vi "HW_Init_Serial_3.vi"(8 "error in":errorcluster, 9 "Acquisition FPS":T2, 10 "Close port? (F)":bool, 11 "VISA resource name":refnum<visa-resource-name>="Tracker") -> (0 "error out":errorcluster, 1 "FPS status":i32=80, 2 "Instrument OK?":bool, 3 "VISA resource name out":refnum<visa-resource-name>, 4 "Init status":T1={"VISA resource name"="", "FW version information"="0.0.0", "Sensor board size"="", "Sync mode status"="0", "FPS status"=0, "Instrument OK?"=FALSE})   [LabVIEW 2018, in "HW Interaction.lvlib"]
uses:
  HW Interaction.lvlib
  SubVi's/Controls/CTL_Acquisition_speed_selector.ctl
  Typedefs/CTL_HW_Init_outcome.ctl
  <vilib>/Utility/error.llb/DialogType.ctl
  Typedefs/CTL_HW_Init_internal_commands.ctl
  <vilib>/Instr/_visa.llb/VISA Set IO Buffer Mask.ctl
  <vilib>/Instr/_visa.llb/VISA Flush IO Buffer Mask.ctl
  <vilib>/Instr/_visa.llb/VISA Configure Serial Port (Instr).vi
  HW_Poll_Tracker_1.x.x.vi
  HW_Poll_Tracker_2.0.3.vi
  HW_Poll_Tracker_2.0.4+.vi
  Common_Resources.lvlib
panel:
  out "FPS setting VISA reply":string
  out "Poll Sync mode status":u32
  in  "FPS setup request":i32=80
  out "Poll Port data status":u32
  out "Port data status":i32=1
  out "Poll Binary":u32
  out "Poll Matrix":u32
  out "Poll Coord":u32
  out "Poll FPS":u32
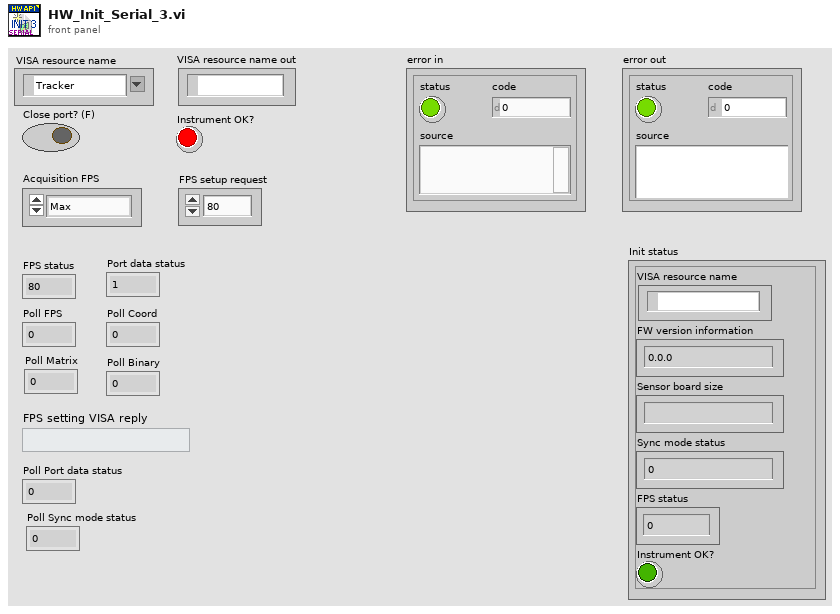
[diagram p1: front panel]
types:
  T1 = typedef "HW Interaction.lvlib/CTL_HW_Init_outcome.ctl" = cluster{"VISA resource name":refnum<visa-resource-name>, "FW version information":string, "Sensor board size":string, "Sync mode status":string, "FPS status":i32, "Instrument OK?":bool}
  T2 = typedef "Common_Resources.lvlib/CTL_Acquisition_speed_selector.ctl" = enum16{"Max", "Optimal", "Eco"}
  T3 = typedef "DialogType.ctl" = u16
  T4 = typedef "HW Interaction.lvlib/CTL_HW_Init_internal_commands.ctl" = cluster{"CMD":enum16{"None", "Exit", "Pause", "Step 1", "Step 2", "Step 3", "Step 4", "Step 5", "Step 6"}, "Payload":variant}
  T5 = enum16{"None", "Exit", "Pause", "Step 1", "Step 2", "Step 3", "Step 4"}
  T6 = enum16{"None", "Exit", "Pause", "Step 1", "Step 2", "Step 3", "Step 4", "Step 5", "Step 6"}
  T7 = typedef "VISA Flush IO Buffer Mask.ctl" = u16
  T8 = typedef "VISA Set IO Buffer Mask.ctl" = u16
  T9 = cluster{"Matrix mode status":string, "Coordinate mode status":string, "Binary mode status":string, "Sensors response":string, "FPS status":i32, "Port data status":i32}
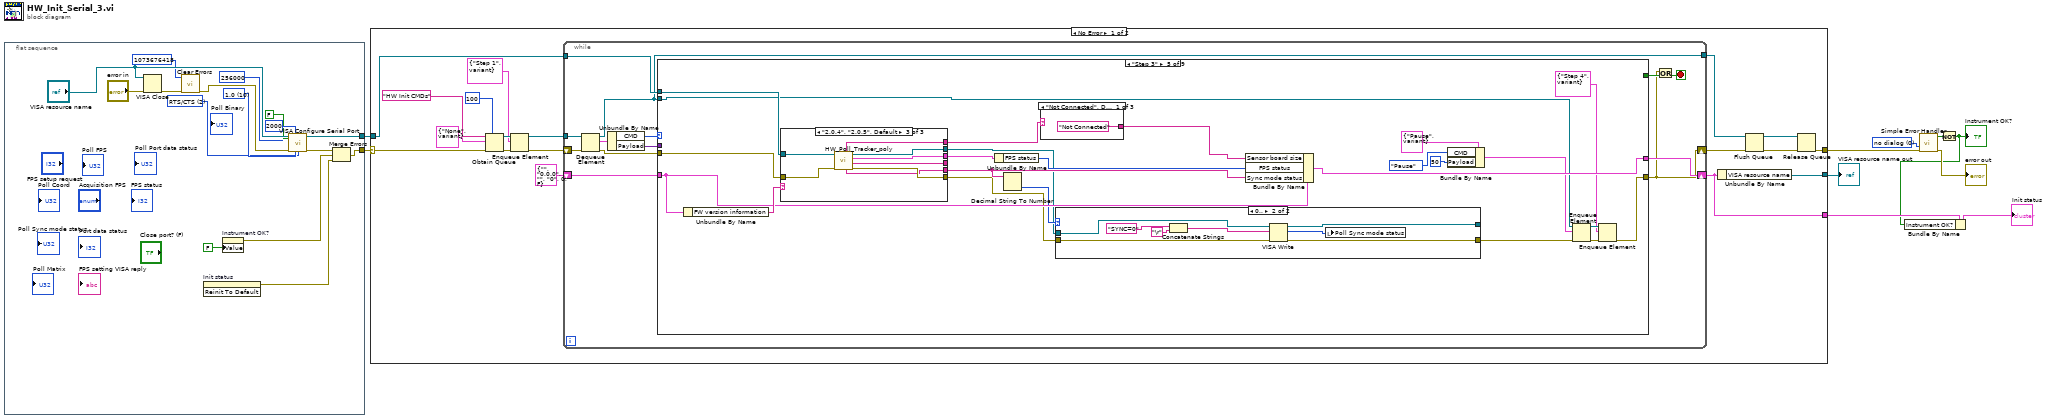
[diagram p0: block diagram]
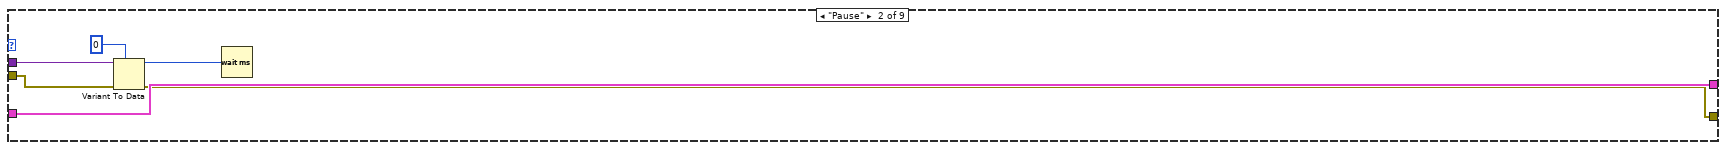
[diagram p3: hidden frame]
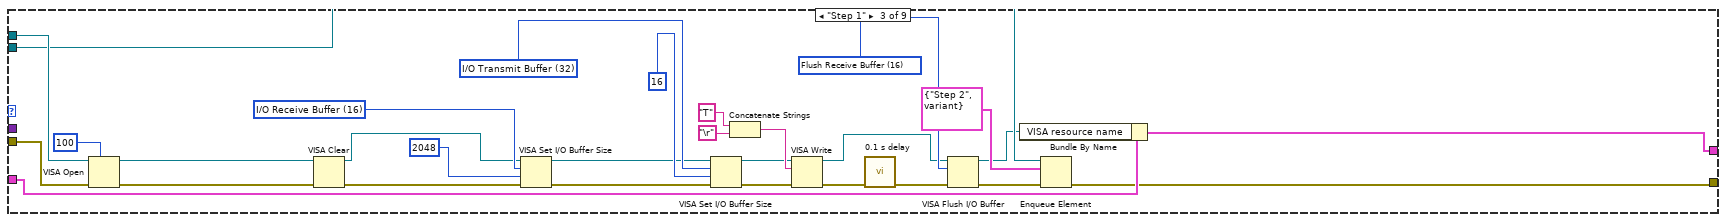
[diagram p4: hidden frame]
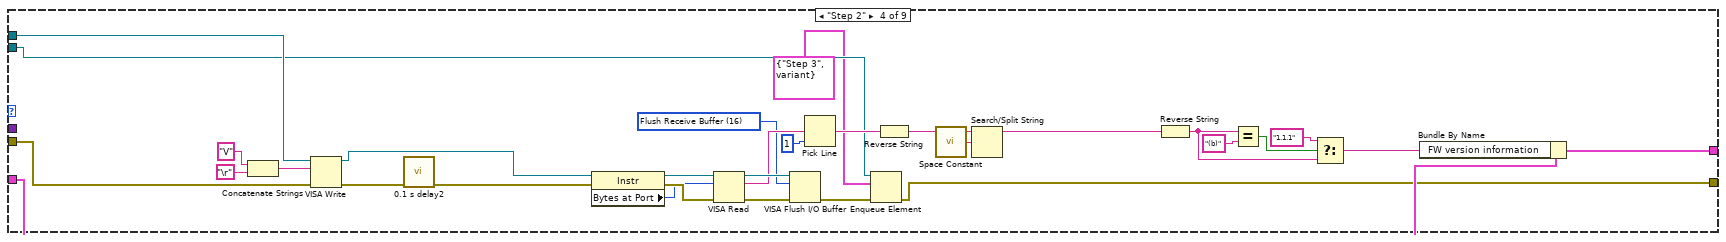
[diagram p5: hidden frame]
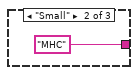
[diagram p6: hidden frame]
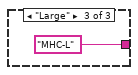
[diagram p7: hidden frame]
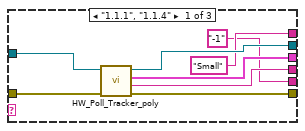
[diagram p9: hidden frame]
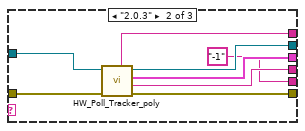
[diagram p10: hidden frame]
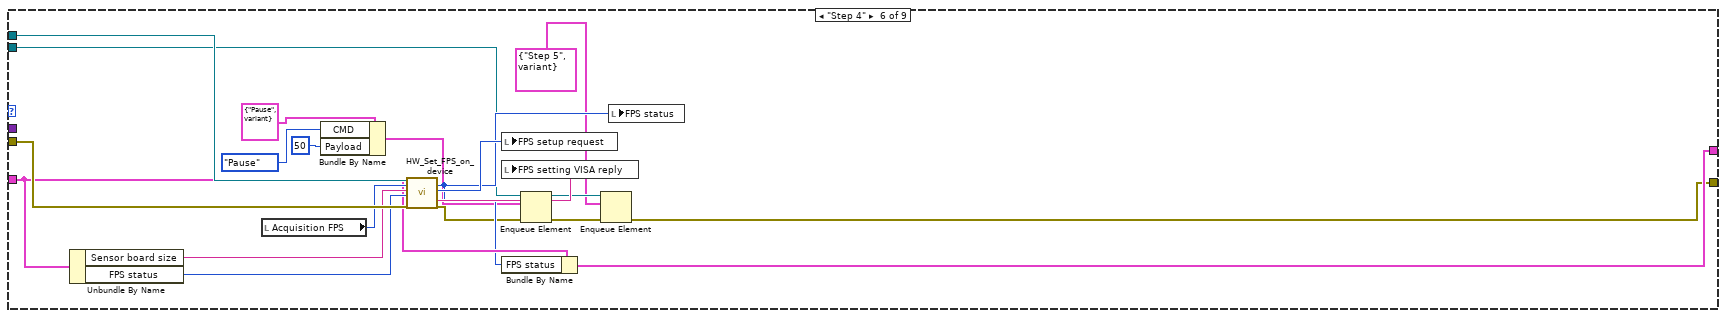
[diagram p11: hidden frame]
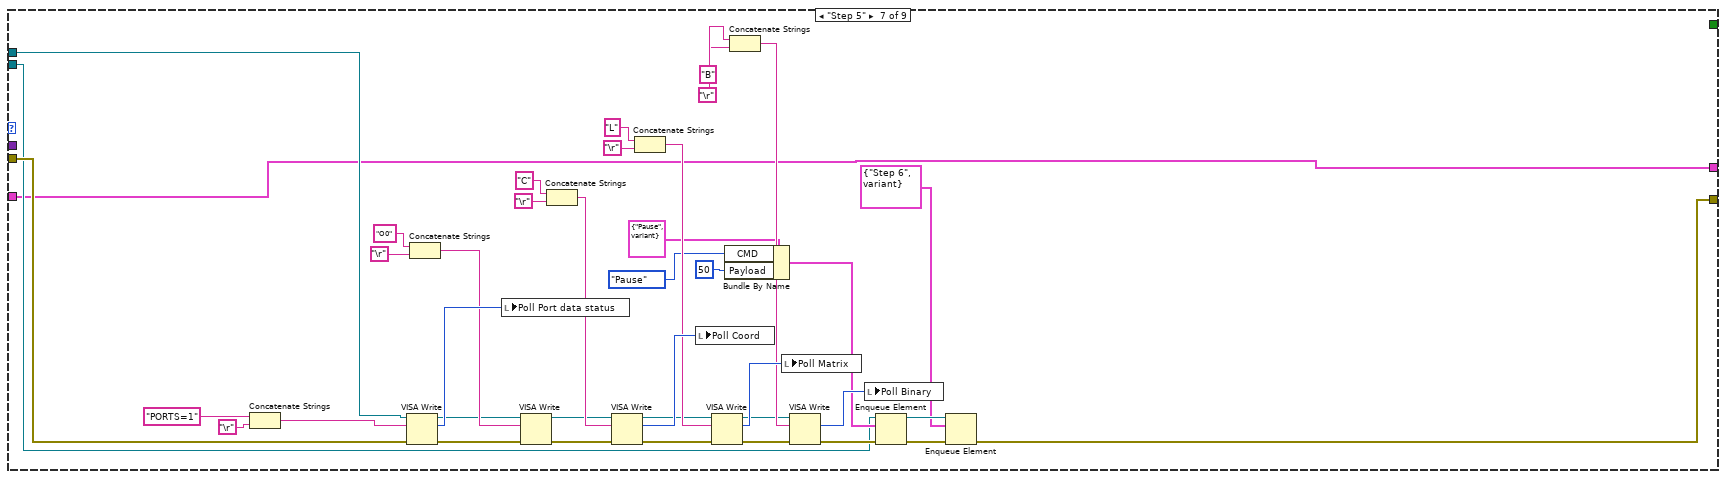
[diagram p12: hidden frame]
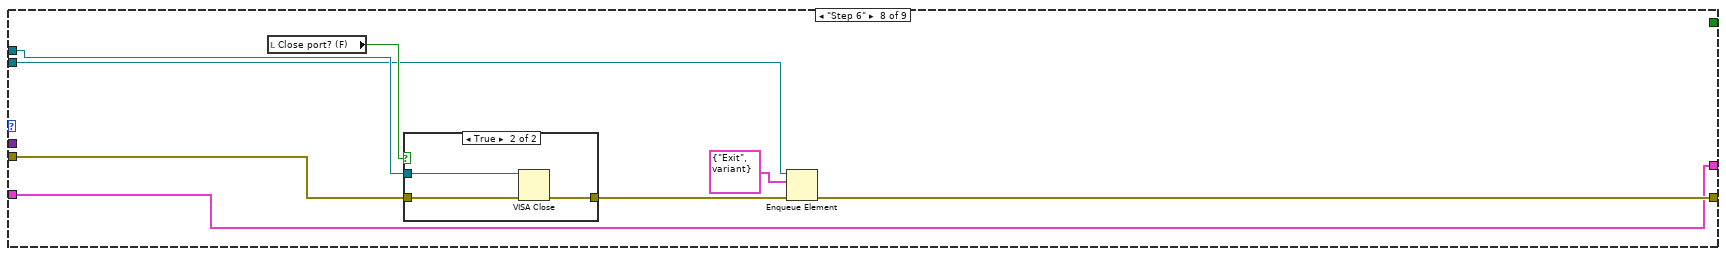
[diagram p13: hidden frame]
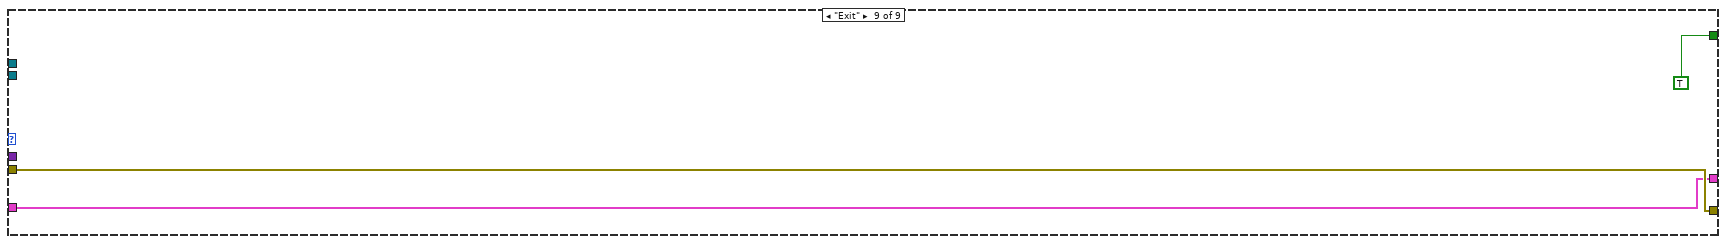
[diagram p15: hidden frame]
diagram:
  w9 = T3 0 items=["no dialog", "OK message", "continue or stop message", "OK message + warnings", "continue/stop + warnings"] ("type of dialog (OK msg:1)")
  n1 = flat-sequence {
    tunnel: [w16] -> w8
    tunnel: [w14] -> w7
    frame #0 {
      w18 = u16 10 items=["1.0"=10, "1.5"=15, "2.0"=20] ("stop bits (10: 1 bit)")
      w17 = u16 2 items=["None", "XON/XOFF", "RTS/CTS", "XON/XOFF & RTS/CTS", "DTR/DSR", "XON/XOFF & DTR/DSR"] ("flow control (0:none)")
      n2 = VISA Close(VISA resource name="VISA resource name", error in (no error)="error in") -> (error out=w24:errorcluster)
      n3 = call <vilib>:"Clear Errors.vi"("error in (no error)"=w24, "specific error code to clear (0: all)"=1073676418) -> ("error out"=w26:errorcluster)  [unwired: 4 in, 1 out]
      n4 = invoke on="Init status" class="Clust (strict)" method="Reinit To Default"() -> (error out=w11:errorcluster)  [unwired: 3 in, 2 out]
      n5 = property on="Instrument OK?" class="Bool (strict)"("Value"=FALSE ("Instrument OK?")) -> (error out=w12:errorcluster)  [unwired: 2 in, 1 out]
      n6 = call-poly "VISA Configure Serial Port"("VISA resource name"="VISA resource name", "timeout (10sec)"=u32 2000, "Enable Termination\nChar (T)"=FALSE ("Enable Termination\nChar (T)"), "baud rate (9600)"=u32 256000, "error in (no error)"=w26, "stop bits (10: 1 bit)"=w18, "flow control (0:none)"=w17) -> ("VISA resource name out"=w16:refnum<visa-resource-name>, "error out"=w15:errorcluster)  [unwired: 7 in]
      n7 = Merge Errors(w15, w12, w11) -> (w14:errorcluster)
    }
  }
  n8 = case shown="No Error" w7 {
    selector: w7 -> [w41 w261]
    tunnel: w8 -> [w44 w262]
    tunnel: [w29 w261] -> w6
    tunnel: [w28 _] -> w5
    tunnel: [w27 w262] -> w4
    frame No Error {
      n9 = Obtain Queue(max queue size (-1, unlimited)=100, name (unnamed)="HW Init CMDs", element data type=T4 {"CMD"=enum."None", "Payload"=variant} ("CMD and payload"), error in (no error)=w41) -> (queue out=w37:refnum<queue>, error out=w38:errorcluster)  [unwired: 1 in, 1 out]
      n10 = Enqueue Element(queue=w37, element=T4 {"CMD"=enum."Step 1", "Payload"=variant}, error in (no error)=w38) -> (queue out=w36:refnum<queue>, error out=w35:errorcluster)  [unwired: 1 in, 1 out]
      n11 = while {
        shift-right: [w45] -> w33
        shift-left: w35 -> [w53]
        tunnel: w44 -> [w56]
        shift-right: [w54] -> w28
        shift-left: T1 {"VISA resource name"="", "FW version information"="0.0.0", "Sensor board size"="", "Sync mode status"="0", "FPS status"=0, "Instrument OK?"=FALSE} ("Init status") -> [w55]
        tunnel: w36 -> [w51]
        tunnel: [w50] -> w32
        stop <- w46 stop-if-true
        n12 = Dequeue Element(queue=w51, error in (no error)=w53) -> (queue out=w50:refnum<queue>, element=w49:T4, error out=w52:errorcluster)  [unwired: 1 in, 1 out]
        n13 = Unbundle By Name(w49) -> ("CMD"=w48:T6, "Payload"=w47:variant)
        n14 = case shown="\"Step 3\"" w48 {
          tunnel: [_ _ _ _ _ _ _ _ TRUE] -> w57
          tunnel: w52 -> [w58 w63 w92 w122 w148 w205 w244 w252 w259]
          tunnel: w56 -> [_ _ w93 w121 w147 w204 w245 w251 _]
          tunnel: w55 -> [w59 w62 w72 w101 w145 w199 w206 w246 w258]
          tunnel: [w59 w62 w67 w99 w144 w198 w206 w246 w258] -> w54
          tunnel: w50 -> [_ _ w70 w97 w137 w195 w208 w250 _]
          tunnel: [w58 w61 w69 w96 w129 w187 w207 w247 w259] -> w45
          tunnel: w47 -> [_ w60 _ _ _ _ _ _ _]
          frame "None", Default {
          }
          frame "Pause" {
            n15 = Variant To Data(error in=w63, type=0, Variant=w60) -> (data=w64:i32, error out=w61:errorcluster)
            n16 = Wait (ms)(milliseconds to wait=w64) -> ()  [unwired: 1 out]
          }
          frame "Step 1" {
            w75 = T7 16 items=["Flush Receive Buffer"=16, "Write Transmit Buffer to Device"=32, "Flush Receive Buffer (No I/O)"=64, "Flush Transmit Buffer"=128] ("Mask")
            w85 = T8 32 items=["I/O Receive Buffer"=16, "I/O Transmit Buffer"=32, "I/O Receive and Transmit Buffer"=48] ("Mask")
            w89 = T8 16 items=["I/O Receive Buffer"=16, "I/O Transmit Buffer"=32, "I/O Receive and Transmit Buffer"=48] ("Mask")
            n17 = VISA Open(timeout (0)=u32 100 ("VISA Open timeout (0)"), error in (no error)=w92, VISA resource name=w93) -> (VISA resource name=w90:refnum<visa-resource-name>, error out=w91:errorcluster)  [unwired: 2 in]
            n18 = VISA Clear(VISA resource name=w90, error in (no error)=w91) -> (VISA resource name out=w86:refnum<visa-resource-name>, error out=w87:errorcluster)
            n19 = VISA Set I/O Buffer Size(VISA resource name=w86, mask (16)=w89, size (4096)=u32 2048, error in (no error)=w87) -> (VISA resource name out=w83:refnum<visa-resource-name>, error out=w82:errorcluster)
            n20 = VISA Set I/O Buffer Size(VISA resource name=w83, mask (16)=w85, size (4096)=u32 16, error in (no error)=w82) -> (VISA resource name out=w77:refnum<visa-resource-name>, error out=w78:errorcluster)
            n21 = Concatenate Strings("T" ("write buffer"), "\r") -> (w81:string)
            n22 = VISA Write(VISA resource name=w77, write buffer=w81, error in (no error)=w78) -> (VISA resource name out=w73:refnum<visa-resource-name>, error out=w76:errorcluster)  [unwired: 1 out]
            n23 = call "0.1 s delay"("error in (no error)"=w76) -> ("error out"=w74:errorcluster)  [unwired: 10 in]
            n24 = VISA Flush I/O Buffer(VISA resource name=w73, mask (16)=w75, error in (no error)=w74) -> (VISA resource name out=w66:refnum<visa-resource-name>, error out=w71:errorcluster)
            n25 = Bundle By Name(cluster=w72, "VISA resource name"=w66) -> (w67:T1)
            n26 = Enqueue Element(queue=w70, element=T4 {"CMD"=enum."Step 2", "Payload"=variant}, error in (no error)=w71) -> (error out=w69:errorcluster)  [unwired: 1 in, 2 out]
          }
          frame "Step 2" {
            w104 = T7 16 items=["Flush Receive Buffer"=16, "Write Transmit Buffer to Device"=32, "Flush Receive Buffer (No I/O)"=64, "Flush Transmit Buffer"=128] ("Mask")
            n27 = Concatenate Strings("V" ("write buffer"), "\r") -> (w125:string)
            n28 = VISA Write(VISA resource name=w121, write buffer=w125, error in (no error)=w122) -> (VISA resource name out=w103:refnum<visa-resource-name>, error out=w120:errorcluster)  [unwired: 1 out]
            n29 = call "0.1 s delay2"("error in (no error)"=w120) -> ("error out"=w102:errorcluster)  [unwired: 10 in]
            n30 = property class="Instr"(reference=w103, error in=w102) -> (reference out=w119:refnum<visa-resource-name>, error out=w118:errorcluster, "Bytes at Port"=w117:u32)
            n31 = VISA Read(VISA resource name=w119, byte count=w117, error in (no error)=w118) -> (VISA resource name out=w115:refnum<visa-resource-name>, read buffer=w114:string, error out=w116:errorcluster)  [unwired: 1 out]
            n32 = VISA Flush I/O Buffer(VISA resource name=w115, mask (16)=w104, error in (no error)=w116) -> (error out=w98:errorcluster)  [unwired: 1 out]
            n33 = Pick Line(multi-line string=w114, line index=1) -> (output string=w113:string)  [unwired: 1 in]
            n34 = Enqueue Element(queue=w97, element=T4 {"CMD"=enum."Step 3", "Payload"=variant}, error in (no error)=w98) -> (error out=w96:errorcluster)  [unwired: 1 in, 2 out]
            n35 = Reverse String(1:w113) -> (0:w112:string)
            n36 = call <vilib>:"Space Constant.vi"() -> ("String"=w111:string)
            n37 = Search/Split String(string=w112, search string/char (-)=w111) -> (substring before match=w110:string)  [unwired: 1 in, 2 out]
            n38 = Reverse String(1:w110) -> (0:w108:string)
            n39 = Equal?(x=w108, y="(b)") -> (x = y?=w109:bool)
            n40 = Select(t="1.1.1", s=w109, f=w108) -> (s? t:f=w100:string)
            n41 = Bundle By Name(cluster=w101, "FW version information"=w100) -> (w99:T1)
          }
          frame "Step 3" {
            n42 = Unbundle By Name(w145) -> ("FW version information"=w146:string)
            n43 = case shown="\"2.0.4\", \"2.0.5\", Default" w146 {
              tunnel: [w169 w174 w183] -> w139
              tunnel: [w168 w172 w180] -> _
              tunnel: w148 -> [w167 w177 w184]
              tunnel: w147 -> [w166 w175 w185]
              tunnel: [w165 w176 w179] -> w138
              tunnel: [w164 w173 w181] -> w143
              tunnel: ["Small" w171 w182] -> w127
              tunnel: ["-1" ("Sync mode status") "-1" ("Sync mode status") w178] -> w140
              frame "1.1.1", "1.1.4" {
                n44 = call-poly "HW_Poll_Tracker_poly.vi"("error in"=w167, "VISA resource name in"=w166) -> ("error out"=w165:errorcluster, "Read buffer"=w168:string, "Parameters output"=w164:T9, "VISA resource name out"=w169:refnum<visa-resource-name>)  [unwired: 6 in]
              }
              frame "2.0.3" {
                n45 = call-poly "HW_Poll_Tracker_poly.vi"("error in"=w177, "VISA resource name in"=w175) -> ("error out"=w176:errorcluster, "Read buffer"=w172:string, "Parameters output"=w173:T9, "VISA resource name out"=w174:refnum<visa-resource-name>, "Sensor board size"=w171:string)  [unwired: 5 in]
              }
              frame "2.0.4", "2.0.5", Default {
                n46 = call-poly "HW_Poll_Tracker_poly.vi"("error in"=w184, "VISA resource name in"=w185) -> ("error out"=w179:errorcluster, "Read buffer"=w180:string, "Parameters output"=w181:T9, "VISA resource name out"=w183:refnum<visa-resource-name>, "Sync mode status"=w178:string, "Sensor board size"=w182:string)  [unwired: 4 in]
              }
            }
            n47 = Unbundle By Name(w143) -> ("FPS status"=w142:i32)
            n48 = Decimal String To Number(string=w140) -> (number=w141:i32)  [unwired: 2 in, 1 out]
            n49 = case shown="\"Not Connected\", Default" w127 {
              tunnel: ["Not Connected" ("f") "MHC" ("x") "MHC-L" ("f")] -> w126
              frame "Not Connected", Default {
              }
              frame "Small" {
              }
              frame "Large" {
              }
            }
            n50 = case shown="0.." w141 {
              tunnel: w139 -> [w153 w160]
              tunnel: w138 -> [w152 w159]
              tunnel: [w152 w158] -> w136
              tunnel: [w153 w157] -> _
              frame -1, Default {
              }
              frame 0.. {
                n51 = Concatenate Strings("SYNC=0" ("write buffer"), "\r") -> (w161:string)
                n52 = VISA Write(VISA resource name=w160, write buffer=w161, error in (no error)=w159) -> (VISA resource name out=w157:refnum<visa-resource-name>, return count=w154:u32, error out=w158:errorcluster)
                n53 = local write "Poll Sync mode status"(w154) -> ()
              }
            }
            n54 = Bundle By Name(cluster=w145, "Sensor board size"=w126, "FPS status"=w142, "Sync mode status"=w140) -> (w144:T1)
            n55 = Bundle By Name(cluster=T4 {"CMD"=enum."Pause", "Payload"=variant} ("element"), "CMD"=T5."Pause", "Payload"=50) -> (w134:T4)
            n56 = Enqueue Element(queue=w137, element=w134, error in (no error)=w136) -> (queue out=w130:refnum<queue>, error out=w131:errorcluster)  [unwired: 1 in, 1 out]
            n57 = Enqueue Element(queue=w130, element=T4 {"CMD"=enum."Step 4", "Payload"=variant}, error in (no error)=w131) -> (error out=w129:errorcluster)  [unwired: 1 in, 2 out]
          }
          frame "Step 4" {
            n58 = Unbundle By Name(w199) -> ("Sensor board size"=w202:string, "FPS status"=w203:i32)
            n59 = local read "Acquisition FPS"() -> (w201:T2)
            n60 = Bundle By Name(cluster=T4 {"CMD"=enum."Pause", "Payload"=variant} ("element"), "CMD"=T5."Pause", "Payload"=50) -> (w190:T4)
            n61 = call "HW_Set_FPS_on_device.vi"("VISA in"=w204, "Desired FPS"=w201, "Sensor board size"=w202, "Current FPS"=w203, "Error in (no error)"=w205) -> ("FPS set on device"=w196:i32, "FPS requested"=w197:i32, "VISA reply"=w200:string, "Error out"=w194:errorcluster)  [unwired: 9 in, 2 out]
            n62 = local write "FPS setup request"(w197) -> ()
            n63 = local write "FPS setting VISA reply"(w200) -> ()
            n64 = Bundle By Name(cluster=w199, "FPS status"=w196) -> (w198:T1)
            n65 = Enqueue Element(queue=w195, element=w190, error in (no error)=w194) -> (queue out=w188:refnum<queue>, error out=w189:errorcluster)  [unwired: 1 in, 1 out]
            n66 = Enqueue Element(queue=w188, element=T4 {"CMD"=enum."Step 5", "Payload"=variant}, error in (no error)=w189) -> (error out=w187:errorcluster)  [unwired: 1 in, 2 out]
            n67 = local write "FPS status"(w196) -> ()
          }
          frame "Step 5" {
            n68 = Concatenate Strings("PORTS=1" ("write buffer"), "\r") -> (w241:string)
            n69 = VISA Write(VISA resource name=w245, write buffer=w241, error in (no error)=w244) -> (VISA resource name out=w235:refnum<visa-resource-name>, return count=w240:u32, error out=w236:errorcluster)
            n70 = Concatenate Strings("O0" ("write buffer"), "\r") -> (w239:string)
            n71 = local write "Poll Port data status"(w240) -> ()
            n72 = VISA Write(VISA resource name=w235, write buffer=w239, error in (no error)=w236) -> (VISA resource name out=w229:refnum<visa-resource-name>, error out=w230:errorcluster)  [unwired: 1 out]
            n73 = Concatenate Strings("C" ("write buffer"), "\r") -> (w233:string)
            n74 = VISA Write(VISA resource name=w229, write buffer=w233, error in (no error)=w230) -> (VISA resource name out=w223:refnum<visa-resource-name>, return count=w234:u32, error out=w224:errorcluster)
            n75 = Concatenate Strings("L" ("write buffer"), "\r") -> (w227:string)
            n76 = local write "Poll Coord"(w234) -> ()
            n77 = VISA Write(VISA resource name=w223, write buffer=w227, error in (no error)=w224) -> (VISA resource name out=w217:refnum<visa-resource-name>, return count=w228:u32, error out=w218:errorcluster)
            n78 = Bundle By Name(cluster=T4 {"CMD"=enum."Pause", "Payload"=variant} ("element"), "CMD"=T5."Pause", "Payload"=50) -> (w216:T4)
            n79 = Concatenate Strings("B" ("write buffer"), "\r") -> (w221:string)
            n80 = local write "Poll Matrix"(w228) -> ()
            n81 = VISA Write(VISA resource name=w217, write buffer=w221, error in (no error)=w218) -> (return count=w222:u32, error out=w209:errorcluster)  [unwired: 1 out]
            n82 = local write "Poll Binary"(w222) -> ()
            n83 = Enqueue Element(queue=w208, element=w216, error in (no error)=w209) -> (queue out=w214:refnum<queue>, error out=w215:errorcluster)  [unwired: 1 in, 1 out]
            n84 = Enqueue Element(queue=w214, element=T4 {"CMD"=enum."Step 6", "Payload"=variant}, error in (no error)=w215) -> (error out=w207:errorcluster)  [unwired: 1 in, 2 out]
          }
          frame "Step 6" {
            n85 = local read "Close port? (F)"() -> (w253:bool)
            n86 = case shown="True" w253 {
              tunnel: w252 -> [w254 w257]
              tunnel: [w254 w256] -> w249
              tunnel: w251 -> [_ w255]
              frame False {
              }
              frame True {
                n87 = VISA Close(VISA resource name=w255, error in (no error)=w257) -> (error out=w256:errorcluster)
              }
            }
            n88 = Enqueue Element(queue=w250, element=T4 {"CMD"=enum."Exit", "Payload"=variant}, error in (no error)=w249) -> (error out=w247:errorcluster)  [unwired: 1 in, 2 out]
          }
          frame "Exit" {
          }
        }
        n89 = Or(x=w45, y=w57) -> (x .or. y?=w46:bool)
      }
      n90 = Unbundle By Name(w28) -> ("VISA resource name"=w27:refnum<visa-resource-name>)
      n91 = Flush Queue(queue=w32, error in (no error)=w33) -> (queue out=w30:refnum<queue>, error out=w31:errorcluster)  [unwired: 1 out]
      n92 = Release Queue(queue=w30, error in (no error)=w31) -> (error out=w29:errorcluster)  [unwired: 1 in, 2 out]
    }
    frame Error {
    }
  }
  "VISA resource name out" <- w4
  n93 = call <vilib>:"Simple Error Handler.vi"("type of dialog (OK msg:1)"=w9, "error in (no error)"=w6) -> ("error?"=w10:bool, "error out"=→"error out":errorcluster)  [unwired: 3 in, 3 out]
  n94 = Not(x=w10) -> (.not. x?=w1:bool)
  "Instrument OK?" <- w1
  n95 = Bundle By Name(cluster=w5, "Instrument OK?"=w1) -> (→"Init status":T1)
